vi "Units Matcher - 25012016.vi"(3 "Math-w/-ch-VarID":string[](array[string]), 4 "Comp IDs":string[](array[string]), 5 "OnlySubstanceUnits":string[](array[string]), 6 "Sp_Id_Arr":string[](array[string]), 7 "Kinetic Laws":string[](array[string])) -> (0 "Math-w/-ch-VarID Output":string[](array[string]), 1 "Output Laws":string[](array[string]))   [LabVIEW 2014]
doc: "This VI checks if the flag hasOnlySubstanceUnits is set to \"false\". If it is, it modify the kinetic laws to set the units appropriately for ODE."
uses:
  <vilib>/regexp/Match Regular Expression.xnode
panel:
  out "before substring":string
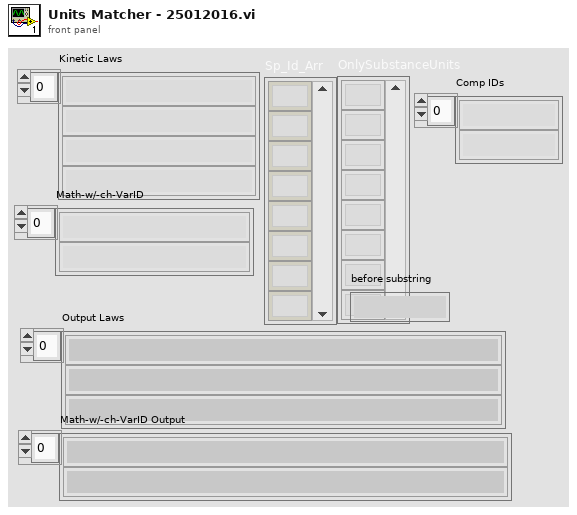
[diagram p1: front panel]
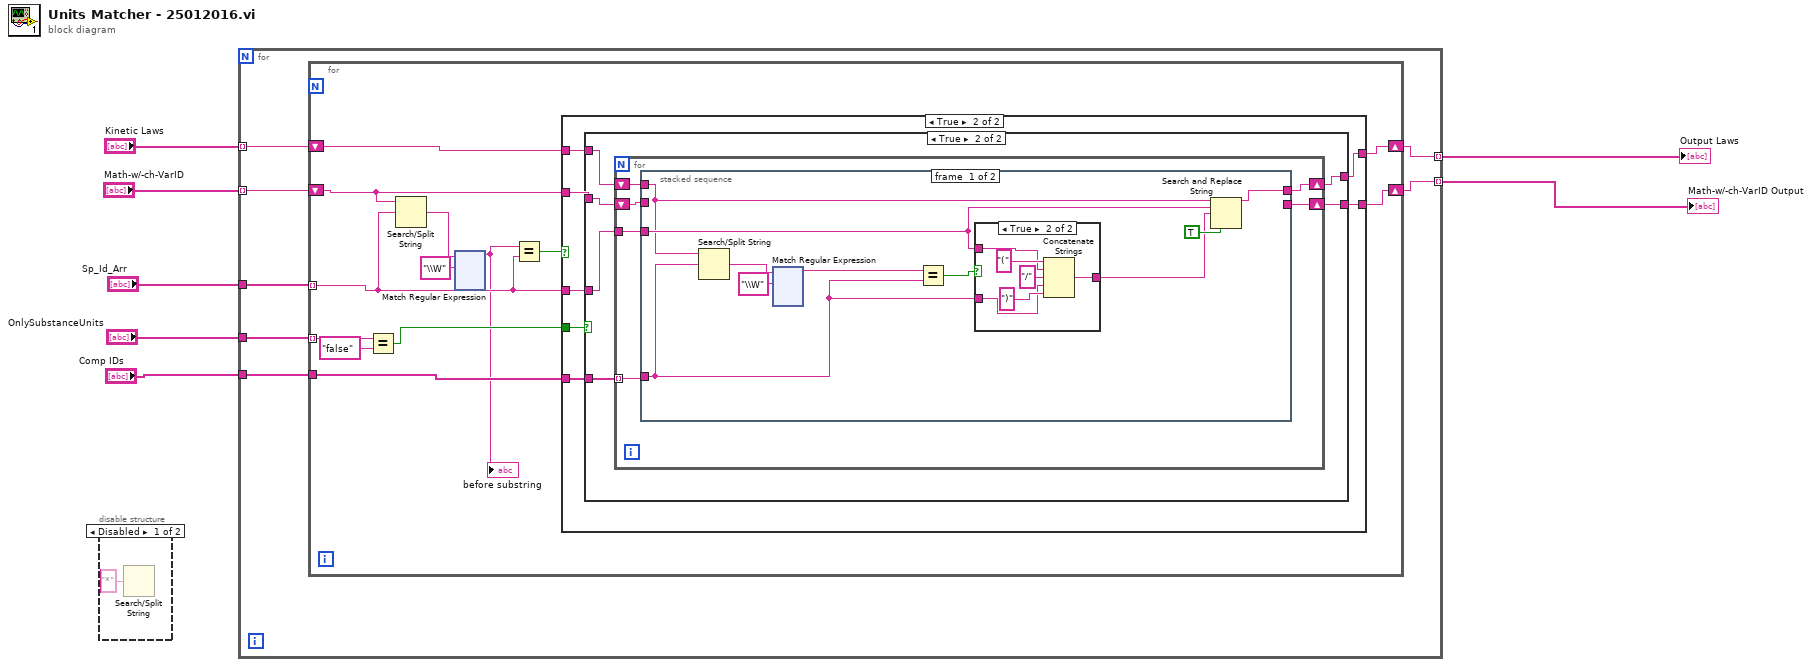
[diagram p0: block diagram]
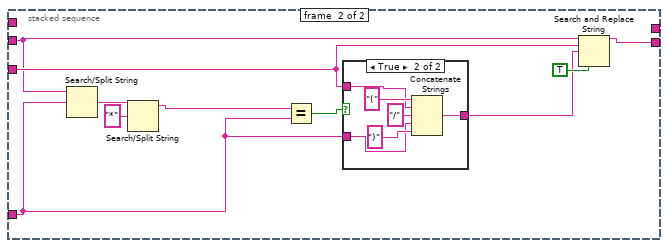
[diagram p6: hidden frame]
diagram:
  n1 = disable-structure shown="Disabled" {
    frame Disabled {
      n2 = Search/Split String(search string/char (-)="*") -> ()  [unwired: 2 in, 3 out]
    }
    frame Enabled {
    }
  }
  n3 = for {
    tunnel: "Sp_Id_Arr" -> [w15]
    tunnel: "OnlySubstanceUnits" -> [w14]
    tunnel: "Comp IDs" -> [w13]
    tunnel: "Kinetic Laws" -> [w12] mode=indexing
    tunnel: [w11] -> w3 mode=indexing
    tunnel: "Math-w/-ch-VarID" -> [w10] mode=indexing
    tunnel: [w9] -> w1 mode=indexing
    n4 = for {
      tunnel: w15 -> [w20] mode=indexing
      tunnel: w14 -> [w28] mode=indexing
      tunnel: w13 -> [w25]
      shift-right: [w23] -> w11
      shift-left: w12 -> [w24]
      shift-right: [w22] -> w9
      shift-left: w10 -> [w21]
      n5 = Equal?(x=w28, y="false") -> (x = y?=w26:bool)
      n6 = Search/Split String(string=w21, search string/char (-)=w20) -> (match + rest of string=w16:string)  [unwired: 1 in, 2 out]
      n7 = xnode "Match Regular Expression"("input string"=w16, "regular expression"="\\W") -> ("before match"=w17:string)  [unwired: 4 in, 4 out]
      "before substring" <- w17
      n8 = Equal?(x=w17, y=w20) -> (x = y?=w19:bool)
      n9 = case shown="True" w19 {
        tunnel: w26 -> [_ w151]
        tunnel: w25 -> [_ w150]
        tunnel: w24 -> [w144 w149]
        tunnel: [w144 w148] -> w23
        tunnel: [w143 w147] -> w22
        tunnel: w21 -> [w143 w146]
        tunnel: w20 -> [_ w145]
        frame False {
        }
        frame True {
          n10 = case shown="True" w151 {
            tunnel: w145 -> [_ w159]
            tunnel: w150 -> [_ w158]
            tunnel: w149 -> [w153 w157]
            tunnel: [w153 w156] -> w148
            tunnel: w146 -> [w152 w155]
            tunnel: [w152 w154] -> w147
            frame False {
            }
            frame True {
              n11 = for {
                tunnel: w159 -> [w165]
                tunnel: w158 -> [w162] mode=indexing
                shift-right: [w164] -> w156
                shift-left: w157 -> [w163]
                shift-right: [w160] -> w154
                shift-left: w155 -> [w161]
                n12 = stacked-sequence {
                  tunnel: w165 -> [w174 w305]
                  tunnel: [w172 _] -> w164
                  tunnel: w163 -> [w171 _]
                  tunnel: w162 -> [w169 w299]
                  tunnel: w161 -> [_ w298]
                  tunnel: [_ w297] -> w160
                  frame #0 {
                    n13 = Search/Split String(string=w171, search string/char (-)=w169) -> (match + rest of string=w167:string)  [unwired: 1 in, 2 out]
                    n14 = xnode "Match Regular Expression"("input string"=w167, "regular expression"="\\W") -> ("before match"=w166:string)  [unwired: 4 in, 4 out]
                    n15 = Equal?(x=w166, y=w169) -> (x = y?=w170:bool)
                    n16 = case shown="True" w170 {
                      tunnel: w174 -> [w290 w295]
                      tunnel: [w290 w292] -> w173
                      tunnel: w169 -> [_ w291]
                      frame False {
                      }
                      frame True {
                        n17 = Concatenate Strings("(" ("string"), w295, "/" ("string"), w291, ")" ("string")) -> (w292:string)
                      }
                    }
                    n18 = Search and Replace String(replace all?=TRUE ("replace all? (F)"), input string=w171, search string=w174, replace string=w173) -> (result string=w172:string)  [unwired: 4 in, 3 out]
                  }
                  frame #1 {
                    n19 = Search/Split String(string=w298, search string/char (-)=w299) -> (match + rest of string=w303:string)  [unwired: 1 in, 2 out]
                    n20 = Search/Split String(string=w303, search string/char (-)="*") -> (substring before match=w301:string)  [unwired: 1 in, 2 out]
                    n21 = Equal?(x=w301, y=w299) -> (x = y?=w300:bool)
                    n22 = case shown="True" w300 {
                      tunnel: w305 -> [w307 w312]
                      tunnel: [w307 w309] -> w304
                      tunnel: w299 -> [_ w308]
                      frame False {
                      }
                      frame True {
                        n23 = Concatenate Strings("(" ("string"), w312, "/" ("string"), w308, ")" ("string")) -> (w309:string)
                      }
                    }
                    n24 = Search and Replace String(replace all?=TRUE ("replace all? (F)"), input string=w298, search string=w305, replace string=w304) -> (result string=w297:string)  [unwired: 4 in, 3 out]
                  }
                }
              }
            }
          }
        }
      }
    }
  }
  "Output Laws" <- w3
  "Math-w/-ch-VarID Output" <- w1
